vi "getCurrents.vi"(0 "Interface in":T1, 11 "error in (no error)":errorcluster) -> (4 "Interface out":T1, 6 "Currents":sgl[](array[numeric]), 8 "TotalCurrent":sgl, 15 "error out":errorcluster)   [LabVIEW 2017, in "BuckBoostInterface.lvlib"]
uses:
  BuckBoostInterface.lvlib
  Interface.ctl
  <instrlib>/_niInstr/Instruction Framework/v1/Host/Instruction Target/niInstr Instruction Target v1 Host.lvclass
  <instrlib>/_niInstr/Instruction Framework/v1/Host/Instruction Framework Context/niInstr Instruction Framework Context v1 Host.lvclass
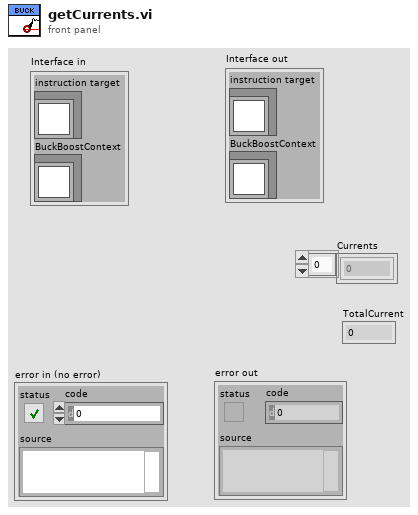
[diagram p1: front panel]
types:
  T1 = typedef "BuckBoostInterface.lvlib/Interface.ctl" = cluster{"instruction target":refnum<class "niInstr Instruction Target v1 Host.lvclass">, "BuckBoostContext":refnum<class "niInstr Instruction Framework Context v1 Host.lvclass">}
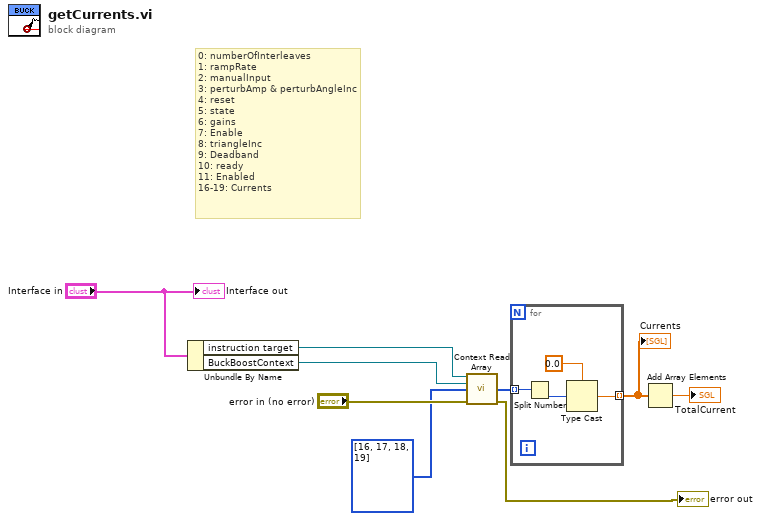
[diagram p0: block diagram]
diagram:
  # "0: numberOfInterleaves\n1: rampRate\n2: manualInput\n3: perturbAmp & perturbAngleInc\n4: reset\n5: state\n6: gains\n7: Enable\n8: triangleInc\n9: Deadband\n10: ready\n11: Enabled\n16-19: Currents"
  n1 = Unbundle By Name("Interface in") -> ("instruction target"=w7:refnum<class "niInstr Instruction Target v1 Host.lvclass">, "BuckBoostContext"=w6:refnum<class "niInstr Instruction Framework Context v1 Host.lvclass">)
  n2 = call <instrlib>:"Context Read Array.vi"("instruction target in"=w7, "context in"=w6, "addresses"=u64[] [16, 17, 18, 19], "error in"="error in (no error)") -> ("data"=w4:u64[], "error out"=→"error out":errorcluster)  [unwired: 8 in, 2 out]
  n3 = for {
    tunnel: w4 -> [w13] mode=indexing
    tunnel: [w10] -> w2 mode=indexing
    n4 = Split Number(x=w13) -> (lo(x)=w12:u32)  [unwired: 1 out]
    n5 = Type Cast(type=sgl 0.0, x=w12) -> (*(type *) &x=w10:sgl)
  }
  "Currents" <- w2
  n6 = Add Array Elements(numeric array=w2) -> (sum=→"TotalCurrent":sgl)
  "Interface out" <- "Interface in"
